vi "DataTranslation_NM2.vi"() -> ()   [LabVIEW 2011]
doc: "This vi will take data with multiple DT boxes for an arbitrary number of channels either differentially or single ended, depending upon how you have wired the boxes up."
uses:
  Controls/DT_Cluster.ctl
  Controls/DT_Mode.ctl
  Controls/Trigger_Mode.ctl
  Globals/Meas_global.vi
  <userlib>/LV-Link3/PolySubVIs/DtOLTimingSetInput.vi
  <userlib>/LV-Link3/PolySubVIs/DtCreateAinChan.vi
  <userlib>/LV-Link3/PolySubVIs/DtCreateCtrRateChan.vi
  <userlib>/LV-Link3/PolySubVIs/DtOLStartNormal.vi
  <userlib>/LV-Link3/PolySubVIs/DtOLReadMultiple2D.vi
  <userlib>/LV-Link3/PolySubVIs/DtOLTriggerDigital.vi
panel:
  out "DAQ Error":errorcluster
  out "Array":T1[](array[typedef])
  out "Clock Task":i32
  out "Waveform Graph":dbl[][](graph)
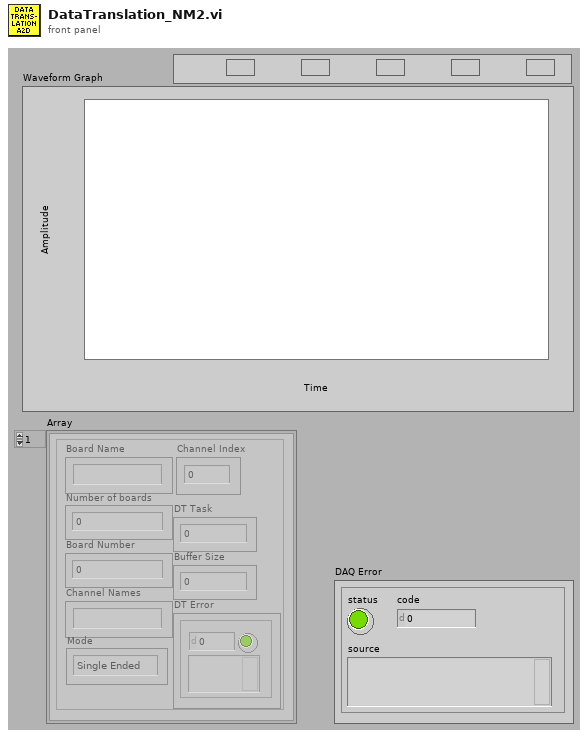
[diagram p1: front panel]
types:
  T1 = typedef "DT_Cluster.ctl" = cluster{"Board Name":string, "Number of boards":u32, "Board Number":u32, "Channel Names":string, "Channel Index":i32[], "DT Task":i32, "DT Error":errorcluster, "Mode":T2, "Buffer Size":u32}
  T2 = typedef "DT_Mode.ctl" = enum16{"Single Ended", "Differential"}
  T3 = typedef "Trigger_Mode.ctl" = enum16{"Free Running", "Start on Trigger", "Trigger Every Block", "Trigger Every Sample"}
  T4 = enum32{"Internal Clock", "External Clock", "No Timing"}
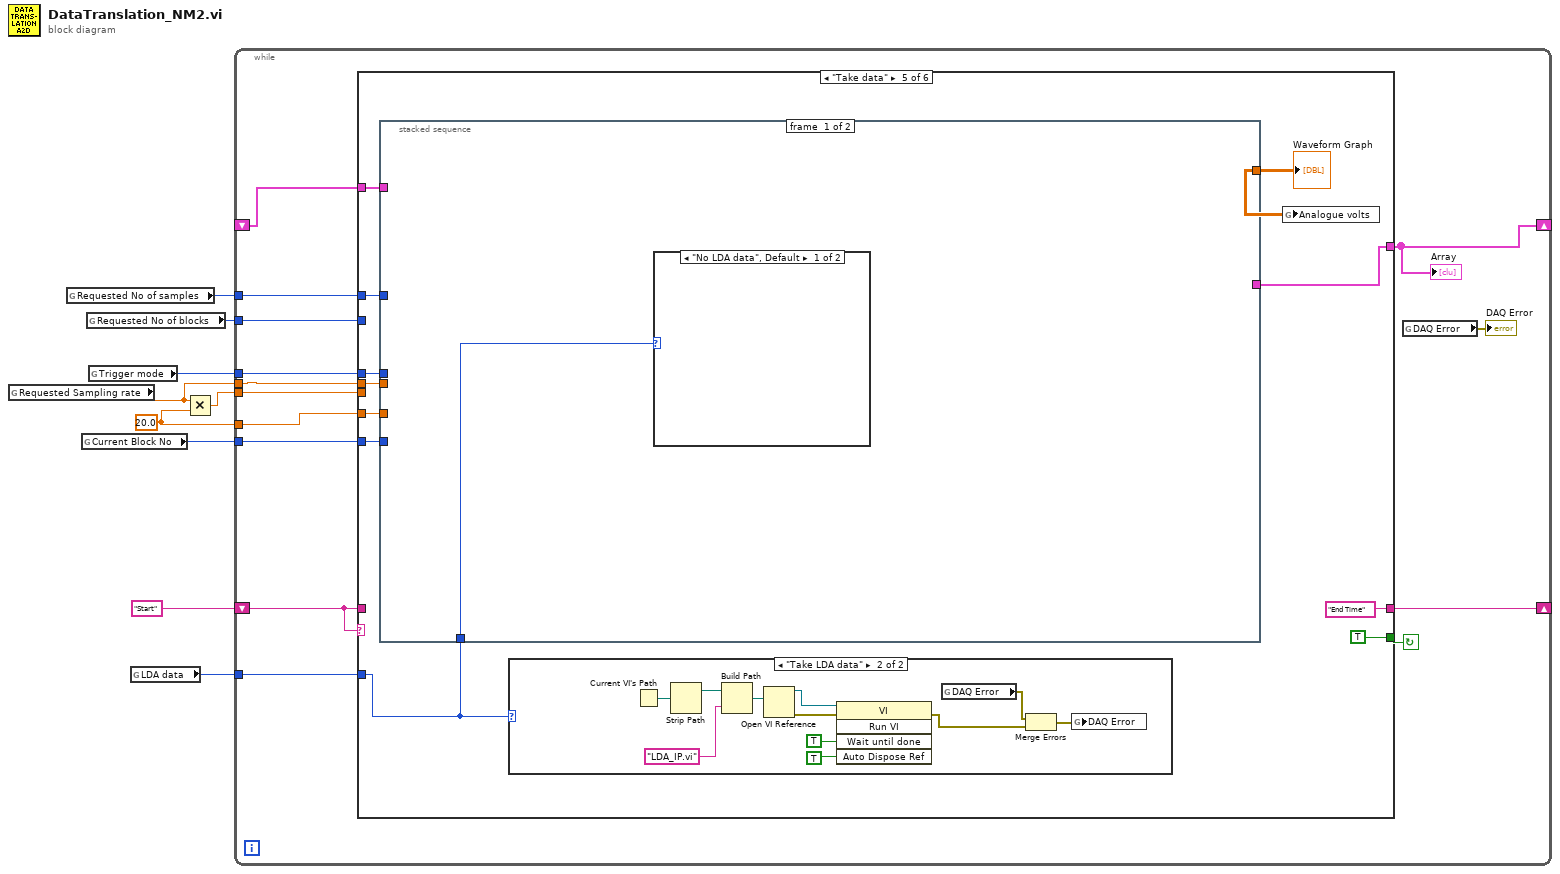
[diagram p0: block diagram]
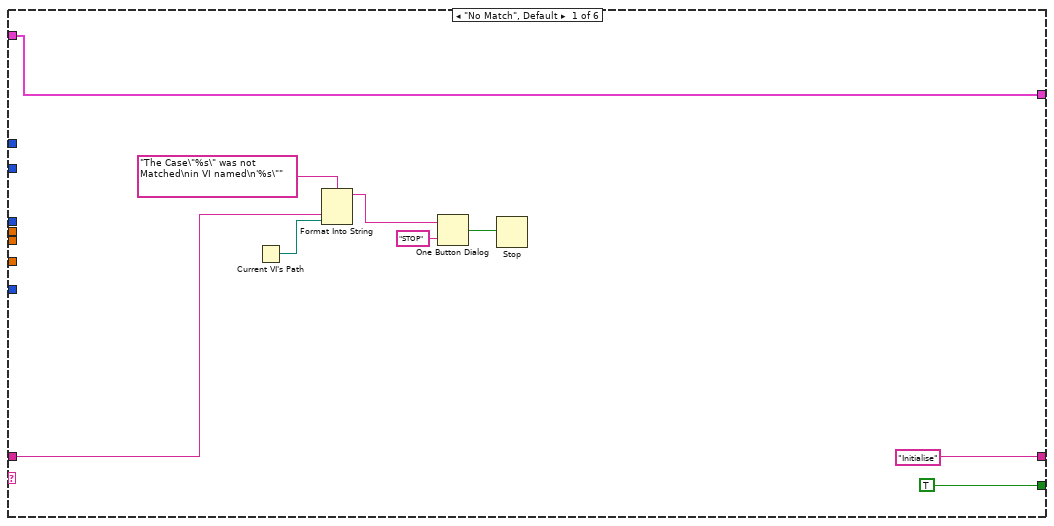
[diagram p2: hidden frame]
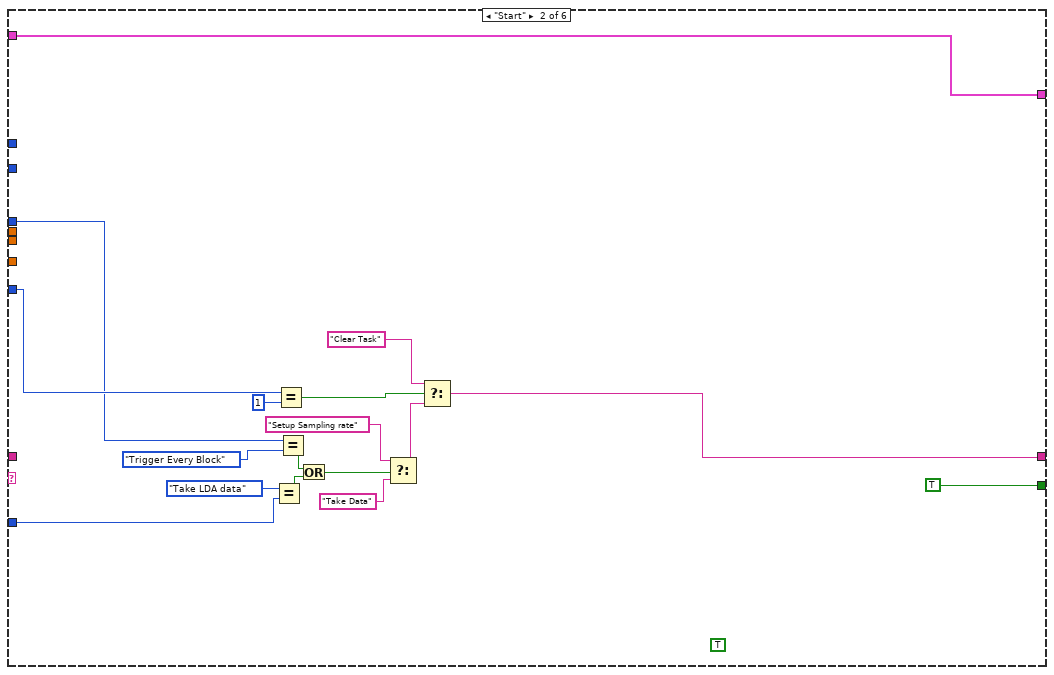
[diagram p3: hidden frame]
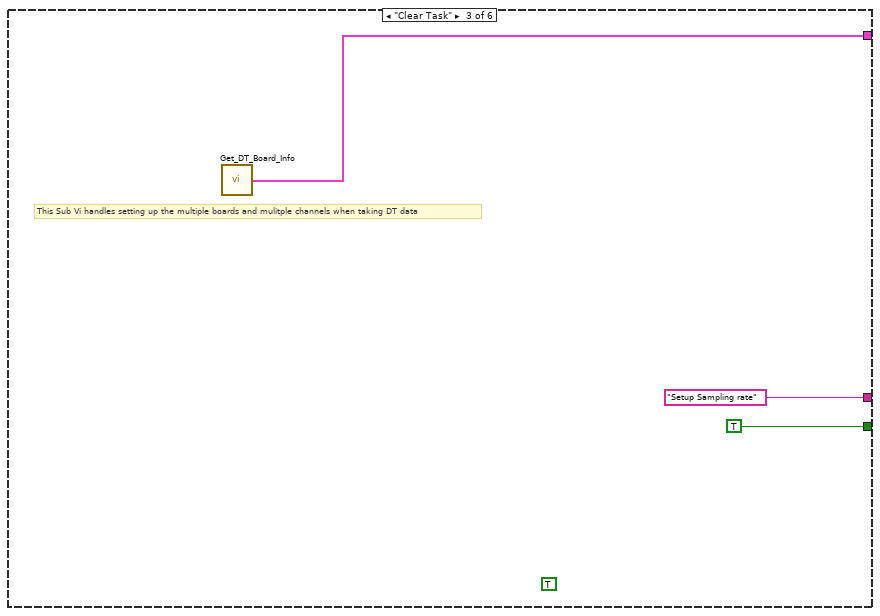
[diagram p4: hidden frame]
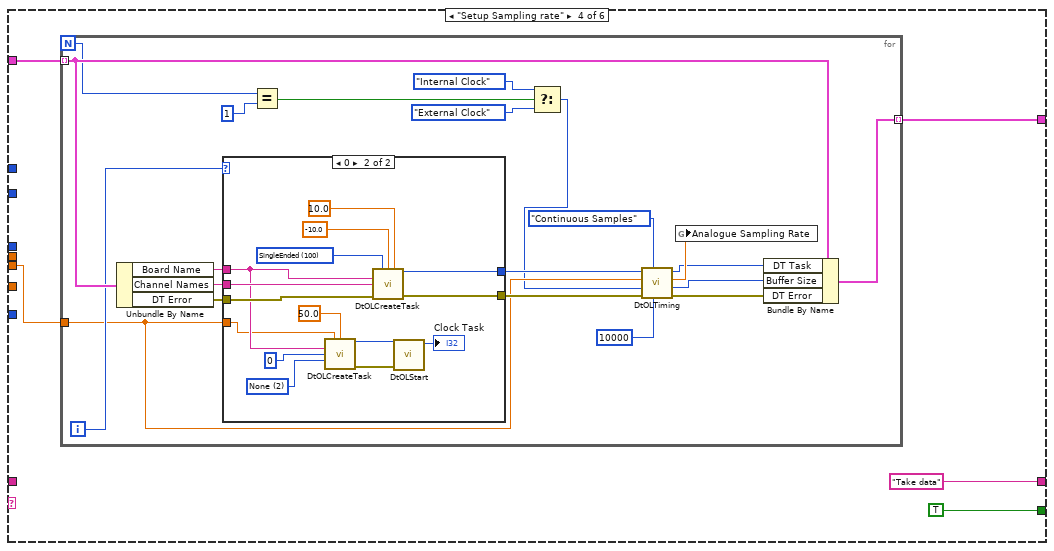
[diagram p5: hidden frame]
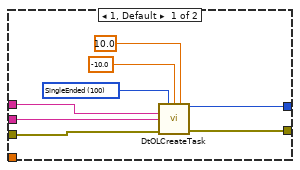
[diagram p6: hidden frame]
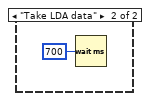
[diagram p8: hidden frame]
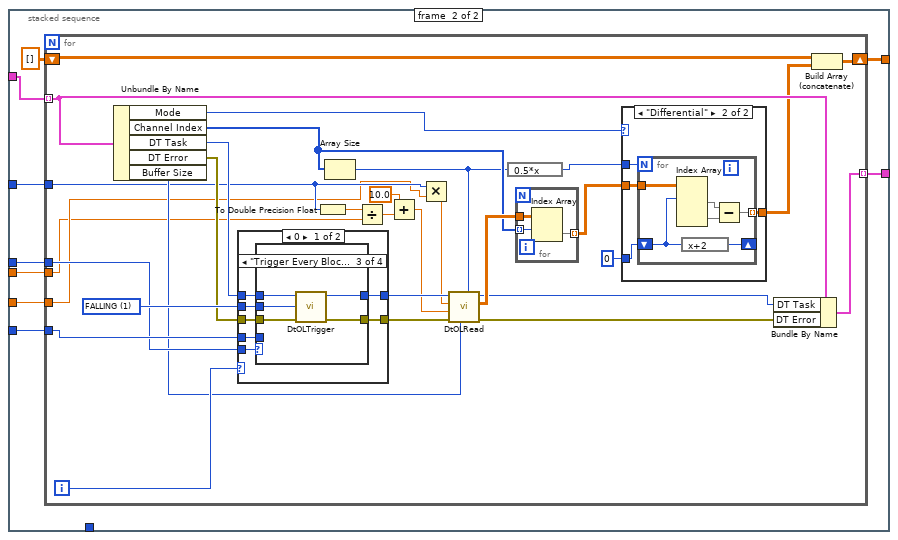
[diagram p9: hidden frame]
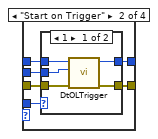
[diagram p12: hidden frame]
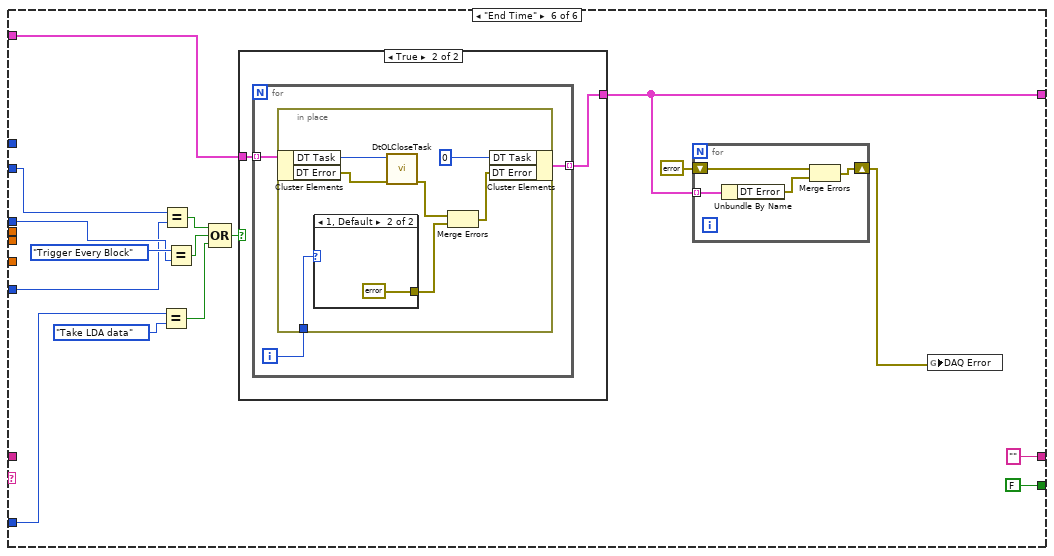
[diagram p16: hidden frame]
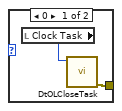
[diagram p18: hidden frame]
diagram:
  w2 = 20.0 ("y")
  n1 = global read "Meas_global.vi" "Requested Sampling rate"() -> (w1:dbl)
  n2 = global read "Meas_global.vi" "Requested No of samples"() -> (w8:i32)
  n3 = global read "Meas_global.vi" "Current Block No"() -> (w6:i32)
  n4 = global read "Meas_global.vi" "Requested No of blocks"() -> (w5:i32)
  n5 = global read "Meas_global.vi" "Trigger mode"() -> (w7:T3)
  n6 = global read "Meas_global.vi" "LDA data"() -> (w4:enum16{"No LDA data", "Take LDA data"})
  n7 = Multiply(x=w1, y=w2) -> (x*y=w3:dbl)
  n8 = while {
    shift-left: "Start" -> [w22]
    shift-right: [w23] -> _
    tunnel: w3 -> [w21]
    tunnel: w8 -> [w20]
    tunnel: w6 -> [w19]
    tunnel: w7 -> [w17]
    tunnel: w5 -> [w16]
    shift-right: [w15] -> _
    shift-left: _ -> [w14]
    tunnel: w4 -> [w12]
    tunnel: w2 -> [w11]
    tunnel: w1 -> [w10]
    stop <- w18 continue-if-true
    n9 = case shown="\"Take data\"" w22 {
      tunnel: ["Initialise" w49 "Setup Sampling rate" "Take data" "End Time" "" ("f")] -> w23
      tunnel: w22 -> [w28 _ _ _ _ _]
      tunnel: w21 -> [_ _ _ w57 _ _]
      tunnel: w20 -> [_ _ _ _ w111 _]
      tunnel: w19 -> [_ w46 _ _ w109 w219]
      tunnel: [TRUE TRUE TRUE TRUE TRUE FALSE] -> w18
      tunnel: w17 -> [_ w44 _ _ w108 w220]
      tunnel: w16 -> [_ _ _ _ _ w221]
      tunnel: w14 -> [w24 w42 _ w54 w107 w217]
      tunnel: [w24 w42 w50 w53 w106 w216] -> w15
      tunnel: w12 -> [_ w41 _ _ w102 w211]
      tunnel: w11 -> [_ _ _ _ w104 _]
      tunnel: w10 -> [_ _ _ _ w103 _]
      frame "No Match", Default {
        n10 = Current VI's Path() -> (path=w27:path)
        n11 = Format Into String(format string="The Case\"%s\" was not Matched\nin VI named\n'%s\"" ("Format String"), w28, w27) -> (resulting string=w31:string)  [unwired: 2 in, 1 out]
        n12 = One Button Dialog(message=w31, button name ("OK")="STOP") -> (true=w29:bool)
        n13 = Stop(stop? (T)=w29) -> ()
      }
      frame "Start" {
        (unwired) TRUE
        n14 = Equal?(x=enum16{"No LDA data", "Take LDA data"}."Take LDA data", y=w41) -> (x = y?=w37:bool)
        n15 = Equal?(x=w46, y=1) -> (x = y?=w39:bool)
        n16 = Equal?(x=w44, y=Trigger_Mode."Trigger Every Block") -> (x = y?=w38:bool)
        n17 = Or(x=w38, y=w37) -> (x .or. y?=w36:bool)
        n18 = Select(t="Setup Sampling rate" ("f"), s=w36, f="Take Data") -> (s? t:f=w33:string)
        n19 = Select(t="Clear Task", s=w39, f=w33) -> (s? t:f=w49:string)
      }
      frame "Clear Task" {
        (unwired) TRUE
        # "This Sub Vi handles setting up the multiple boards and mulitple channels when taking DT data"
        n20 = call "Get_DT_Board_Info.vi"() -> ("DT Cluster Array"=w50:T1[])  [unwired: 5 in]
      }
      frame "Setup Sampling rate" {
        n21 = for {
          N -> [w63]
          tunnel: w57 -> [w64]
          tunnel: w54 -> [w71] mode=indexing
          tunnel: [w70] -> w53 mode=indexing
          i -> [w65]
          n22 = Unbundle By Name(w71) -> ("Board Name"=w74:string, "Channel Names"=w73:string, "DT Error"=w72:errorcluster)
          n23 = case shown="0" w65 {
            tunnel: [w86 w101] -> w77
            tunnel: [w85 w100] -> w76
            tunnel: w74 -> [w84 w94]
            tunnel: w73 -> [w83 w99]
            tunnel: w72 -> [w82 w98]
            tunnel: w64 -> [_ w87]
            frame 1, Default {
              w79 = 100 items=["SingleEnded"=100, "Differential"=101] ("Channel Type")
              n24 = call-poly <userlib>:"DtOLCreateTask.vi"("Channel Type"=w79, "Range Min"=-10.0, "Range Max"=10.0, "Board Name"=w84, "Channel"=w83, "error in (no error)"=w82) -> ("Task out"=w85:i32, "error out"=w86:errorcluster)  [unwired: 7 in, 1 out]
            }
            frame 0 {
              w92 = 2 items=["LowLevel", "HighLevel", "None"] ("Gate Type")
              w95 = 100 items=["SingleEnded"=100, "Differential"=101] ("Channel Type")
              n25 = call-poly <userlib>:"DtOLCreateTask.vi"("Requested\nFrequency (Hz)"=w87, "Duty Cycle"=50.0, "Board Name"=w94, "Counter Num"=u32 0, "Gate Type"=w92) -> ("Task out"=w89:i32, "error out"=w90:errorcluster)  [unwired: 8 in, 1 out]
              n26 = call-poly <userlib>:"DtOLCreateTask.vi"("Channel Type"=w95, "Range Min"=-10.0, "Range Max"=10.0, "Board Name"=w94, "Channel"=w99, "error in (no error)"=w98) -> ("Task out"=w100:i32, "error out"=w101:errorcluster)  [unwired: 7 in, 1 out]
              n27 = call-poly <userlib>:"DtOLStart.vi"("error in (no error)"=w90, "Task in"=w89) -> ("Task out"=→"Clock Task":i32)  [unwired: 8 in, 1 out]
            }
          }
          n28 = Equal?(x=w63, y=1) -> (x = y?=w59:bool)
          n29 = Select(t=T4."Internal Clock" ("Timing"), s=w59, f=T4."External Clock" ("Timing")) -> (s? t:f=w58:T4)
          n30 = call-poly <userlib>:"DtOLTiming.vi"("Num Buffers"=u32 10000, "Sample Mode"=enum16{"Finite Samples", "Continuous Samples"}."Continuous Samples", "error in (no error)"=w77, "Timing"=w58, "Sample Freq (Hz)"=w64, "Task in"=w76) -> ("error out"=w66:errorcluster, "Buffer Size"=w67:u32, "Actual Sample Freq"=w69:dbl, "Task out"=w68:i32)  [unwired: 2 in]
          n31 = global write "Meas_global.vi" "Analogue Sampling Rate"(w69) -> ()
          n32 = Bundle By Name(cluster=w71, "DT Task"=w68, "Buffer Size"=w67, "DT Error"=w66) -> (w70:T1)
        }
      }
      frame "Take data" {
        n33 = stacked-sequence {
          tunnel: w111 -> [_ w134]
          tunnel: w109 -> [_ w133]
          tunnel: w108 -> [_ w132]
          tunnel: w107 -> [_ w131]
          tunnel: [_ w130] -> w106
          tunnel: [_ w128] -> w105
          tunnel: w104 -> [_ w127]
          tunnel: w103 -> [_ w126]
          tunnel: w102 -> [w124 _]
          frame #0 {
            n34 = case shown="\"No LDA data\", Default" w124 {
              frame "No LDA data", Default {
              }
              frame "Take LDA data" {
                n35 = Wait (ms)(milliseconds to wait=u32 700) -> ()  [unwired: 1 out]
              }
            }
          }
          frame #1 {
            n36 = for {
              tunnel: w134 -> [w138]
              tunnel: w133 -> [w163]
              tunnel: w132 -> [w162]
              tunnel: w131 -> [w158] mode=indexing
              tunnel: [w157] -> w130 mode=indexing
              shift-right: [w154] -> w128
              shift-left: dbl[][] [] -> [w153]
              tunnel: w127 -> [w137]
              tunnel: w126 -> [w135]
              i -> [w148]
              w164 = 1 items=["RISING", "FALLING"] ("External Trigger Polarity")
              n37 = Unbundle By Name(w158) -> ("Mode"=w144:T2, "Channel Index"=w155:i32[], "DT Task"=w161:i32, "DT Error"=w160:errorcluster, "Buffer Size"=w140:u32)
              n38 = case shown="0" w148 {
                tunnel: [w183 w207] -> w165
                tunnel: w164 -> [w182 _]
                tunnel: w163 -> [w181 _]
                tunnel: w162 -> [w180 _]
                tunnel: w161 -> [w179 w207]
                tunnel: w160 -> [w178 w206]
                tunnel: [w177 w206] -> w159
                frame 0 {
                  n39 = case shown="\"Trigger Every Block\"" w180 {
                    tunnel: [w185 w189 w201 w205] -> w183
                    tunnel: w179 -> [w185 w190 w203 w205]
                    tunnel: w181 -> [_ w191 _ _]
                    tunnel: w182 -> [_ w188 w202 _]
                    tunnel: w178 -> [w184 w187 w200 w204]
                    tunnel: [w184 w186 w199 w204] -> w177
                    frame "Free Running" {
                    }
                    frame "Start on Trigger" {
                      n40 = case shown="1" w191 {
                        tunnel: w190 -> [w196 w198]
                        tunnel: w187 -> [w195 w197]
                        tunnel: [w193 w198] -> w189
                        tunnel: [w194 w197] -> w186
                        tunnel: w188 -> [w192 _]
                        frame 1 {
                          n41 = call-poly <userlib>:"DtOLTrigger.vi"("error in (no error)"=w195, "External Trigger Polarity"=w192, "Task in"=w196) -> ("error out"=w194:errorcluster, "Task out"=w193:i32)  [unwired: 7 in]
                        }
                        frame 2, Default {
                        }
                      }
                    }
                    frame "Trigger Every Block" {
                      n42 = call-poly <userlib>:"DtOLTrigger.vi"("error in (no error)"=w200, "External Trigger Polarity"=w202, "Task in"=w203) -> ("error out"=w199:errorcluster, "Task out"=w201:i32)  [unwired: 7 in]
                    }
                    frame "Trigger Every Sample" {
                    }
                  }
                }
                frame 1, Default {
                }
              }
              n43 = To Double Precision Float(number=w138) -> (double precision float=w152:dbl)
              n44 = Array Size(array=w155) -> (size(s)=w142:i32)
              n45 = Divide(x=w152, y=w135) -> (x/y=w151:dbl)
              n46 = Add(x=10.0, y=w151) -> (x+y=w149:dbl)
              n47 = Multiply(x=w138, y=w137) -> (x*y=w136:dbl)
              n48 = call-poly <userlib>:"DtOLRead.vi"("Number Chan to Read"=w142, "Buffer size"=w140, "error in (no error)"=w159, "Timeout"=w149, "Samples Per Channel"=w136, "Task in"=w165) -> ("error out"=w139:errorcluster, "2D Data out"=w156:dbl[][], "Task out"=w147:i32)  [unwired: 1 in, 2 out]
              n49 = expression code="0.5*x"(w142) -> (w141:i32)
              n50 = for {
                tunnel: w155 -> [w210] mode=indexing
                tunnel: w156 -> [w209]
                tunnel: [w208] -> w146 mode=indexing
                n51 = Index Array(array=w209, index (row)=w210) -> (element=w208:dbl[])  [unwired: 1 in]
              }
              n52 = case shown="\"Differential\"" w144 {
                tunnel: w146 -> [w166 w170]
                tunnel: [w166 w169] -> w145
                tunnel: 0 ("size(s)") -> [_ w168]
                tunnel: w141 -> [_ w167]
                frame "Single Ended", Default {
                }
                frame "Differential" {
                  n53 = for {
                    N: w167 -> [_]
                    tunnel: w170 -> [w176]
                    shift-right: [w175] -> _
                    shift-left: w168 -> [w174]
                    tunnel: [w172] -> w169 mode=indexing
                    n54 = Index Array(array=w176, index (row) #1=w174) -> (element #1=w171:dbl[], element #2=w173:dbl[])  [unwired: 3 in]
                    n55 = expression code="x+2"(w174) -> (w175:i32)
                    n56 = Subtract(x=w171, y=w173) -> (x-y=w172:dbl[])
                  }
                }
              }
              n57 = Bundle By Name(cluster=w158, "DT Task"=w147, "DT Error"=w139) -> (w157:T1)
              n58 = Build Array (concatenate)(w153, w145) -> (w154:dbl[][])
            }
          }
        }
        "Waveform Graph" <- w105
        n59 = case shown="\"Take LDA data\"" w102 {
          frame "No LDA data", Default {
          }
          frame "Take LDA data" {
            n60 = Current VI's Path() -> (path=w117:path)
            n61 = Strip Path(path=w117) -> (stripped path=w113:path)  [unwired: 1 out]
            n62 = Build Path(base path=w113, name or relative path="LDA_IP.vi") -> (appended path=w118:path)
            n63 = Open VI Reference(vi path=w118) -> (vi reference=w121:refnum<vi>, error out=w122:errorcluster)  [unwired: 5 in]
            n64 = invoke class="VI" method="Run VI"(reference=w121, error in=w122, "Wait until done"=TRUE ("Wait Until Done"), "Auto Dispose Ref"=TRUE ("Wait until done")) -> (error out=w115:errorcluster)  [unwired: 1 in, 4 out]
            n65 = global read "Meas_global.vi" "DAQ Error"() -> (w116:errorcluster)
            n66 = Merge Errors(w116, w115) -> (w114:errorcluster)
            n67 = global write "Meas_global.vi" "DAQ Error"(w114) -> ()
          }
        }
        n68 = global write "Meas_global.vi" "Analogue volts"(w105) -> ()
      }
      frame "End Time" {
        n69 = Equal?(x=w211, y=enum16{"No LDA data", "Take LDA data"}."Take LDA data") -> (x = y?=w213:bool)
        n70 = Equal?(x=w221, y=w219) -> (x = y?=w223:bool)
        n71 = Equal?(x=Trigger_Mode."Trigger Every Block", y=w220) -> (x = y?=w222:bool)
        n72 = Compound Arithmetic op=OR(w223, w222, w213) -> (w218:bool)
        n73 = case shown="True" w218 {
          tunnel: w217 -> [w231 w233]
          tunnel: [w231 w232] -> w216
          frame False {
          }
          frame True {
            n74 = for {
              tunnel: w233 -> [w236] mode=indexing
              tunnel: [w235] -> w232 mode=indexing
              i -> [w234]
              n75 = in-place {
                in-place-border: w234 -> [w237]
                n76 = in-place-cluster #1(w236) -> ("DT Task"=w243:i32, "DT Error"=w242:errorcluster)
                n77 = case shown="1, Default" w237 {
                  tunnel: [w244 errorcluster {"status"=FALSE, "code"=0, "source"=""} ("Error Out")] -> w241
                  frame 0 {
                    n78 = local read "Clock Task"() -> (w245:i32)
                    n79 = call <userlib>:"DtOLCloseTask.vi"("Task in"=w245) -> ("Error Out"=w244:errorcluster)  [unwired: 10 in]
                  }
                  frame 1, Default {
                  }
                }
                n80 = call <userlib>:"DtOLCloseTask.vi"("Error in"=w242, "Task in"=w243) -> ("Error Out"=w240:errorcluster)  [unwired: 9 in]
                n81 = Merge Errors(w240, w241) -> (w239:errorcluster)
                n82 = in-place-cluster #1("DT Task"=0, "DT Error"=w239) -> (w235:T1)
              }
            }
          }
        }
        n83 = for {
          tunnel: w216 -> [w230] mode=indexing
          shift-right: [w227] -> w212
          shift-left: errorcluster {"status"=FALSE, "code"=0, "source"=""} ("error IO") -> [w228]
          n84 = Unbundle By Name(w230) -> ("DT Error"=w229:errorcluster)
          n85 = Merge Errors(w228, w229) -> (w227:errorcluster)
        }
        n86 = global write "Meas_global.vi" "DAQ Error"(w212) -> ()
      }
    }
    "Array" <- w15
    n87 = global read "Meas_global.vi" "DAQ Error"() -> (→"DAQ Error":errorcluster)
  }
